vi "Replace Color.vi"(4 "Use New Fill Algorithm? (F)":bool, 5 "Swap Out White":bool, 6 "Points In":i32[][](array[numeric]), 7 "New Color":u32(colorbox), 8 "5 Pixels":i32[][](array[numeric]), 9 "Ref Color":u32, 10 "U32 color":u32[](array[numeric]), 11 "Rectangle":T1={"left"=0, "top"=0, "right"=32, "bottom"=32}) -> (3 "RGB out":u8[](array[numeric]))   [LabVIEW 2021, in "lv_icon.lvlib"]
doc: "Fill all neightbouring pixels with a certain color based on the incoming start coordinates."
uses:
  lv_icon.lvlib
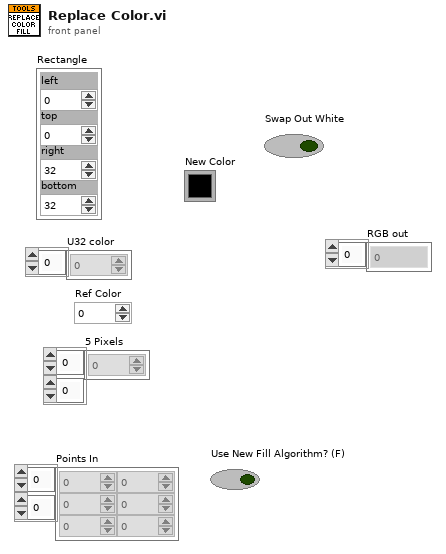
[diagram p1: front panel]
types:
  T1 = cluster{"left":i16, "top":i16, "right":i16, "bottom":i16}
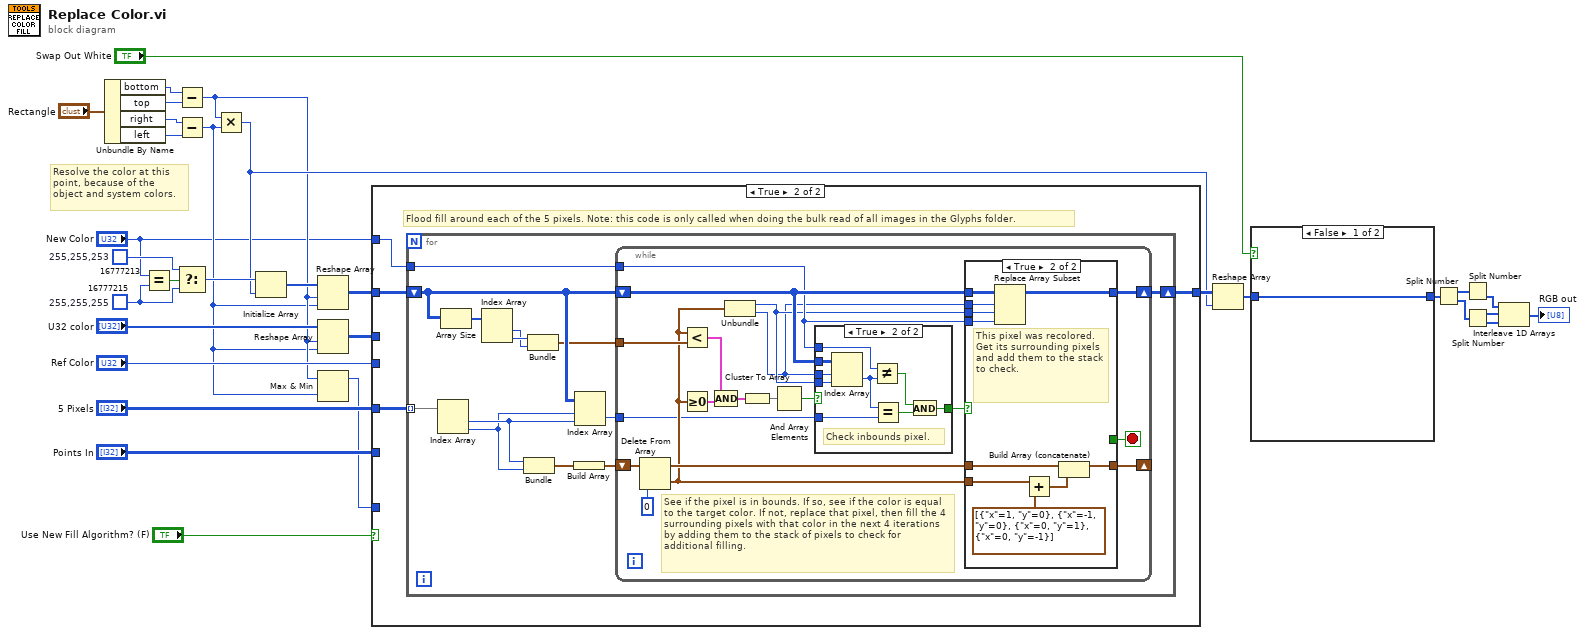
[diagram p0: block diagram]
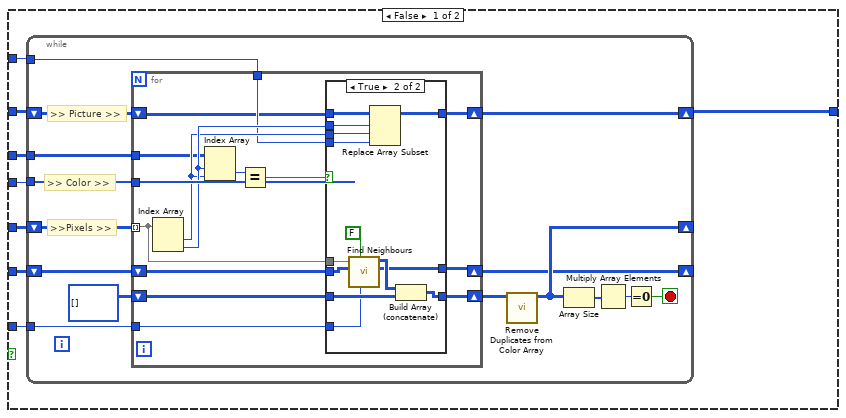
[diagram p2: hidden frame]
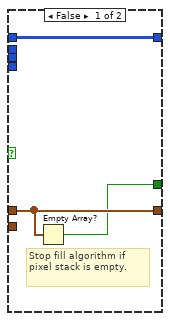
[diagram p5: hidden frame]
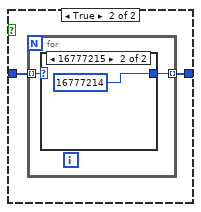
[diagram p6: hidden frame]
diagram:
  w7 = u32 16777213  # 255,255,253
  w6 = u32 16777215  # 255,255,255
  # "Resolve the color at this\npoint, because of the\nobject and system colors."
  n1 = Unbundle By Name("Rectangle") -> ("bottom"=w13:i16, "top"=w14:i16, "right"=w15:i16, "left"=w16:i16)
  n2 = Equal?(x="New Color", y=w6) -> (x = y?=w8:bool)
  n3 = Subtract(x=w13, y=w14) -> (x-y=w11:i16)
  n4 = Subtract(x=w15, y=w16) -> (x-y=w10:i16)
  n5 = Select(t=w7, s=w8, f=w6) -> (s? t:f=w18:u32)
  n6 = Multiply(x=w11, y=w10) -> (x*y=w12:i16)
  n7 = Initialize Array(w18, w12) -> (w28:u32[])
  n8 = Reshape Array(w28, w11, w10) -> (w30:u32[][])
  n9 = Reshape Array("U32 color", w11, w10) -> (w29:u32[][])
  n10 = Max & Min(x=w11, y=w10) -> (max(x,y)=w9:i16)  [unwired: 1 out]
  n11 = case shown="True" "Use New Fill Algorithm? (F)" {
    tunnel: "5 Pixels" -> [w40 w87]
    tunnel: w30 -> [w39 w90]
    tunnel: w29 -> [w38 _]
    tunnel: [w37 w89] -> w27
    tunnel: "Points In" -> [w36 _]
    tunnel: "Ref Color" -> [w35 _]
    tunnel: w9 -> [w34 _]
    tunnel: "New Color" -> [w33 w88]
    frame False {
      n12 = while {
        tunnel: w35 -> [w55]
        tunnel: w33 -> [w53]
        shift-right: [w48] -> _
        shift-left: w40 -> [w43]
        shift-right: [w41] -> w37
        shift-left: w39 -> [w47]
        tunnel: w38 -> [w46]
        shift-right: [w45] -> _
        shift-left: w36 -> [w44]
        tunnel: w34 -> [w42]
        stop <- w51 stop-if-true
        # ">> Picture >>"
        # ">>Pixels >>"
        # ">> Color >>"
        n13 = for {
          tunnel: w43 -> [w68] mode=indexing
          tunnel: w55 -> [w70]
          shift-right: [w67] -> w49
          shift-left: i32[][] [] -> [w66]
          tunnel: w53 -> [w62]
          tunnel: w46 -> [w60]
          shift-right: [w56] -> w41
          shift-left: w47 -> [w61]
          shift-right: [w58] -> w45
          shift-left: w44 -> [w59]
          tunnel: w42 -> [w57]
          n14 = Index Array(array=w68) -> (element #1=w63:i32, element #2=w64:i32)  [unwired: 2 in]
          n15 = Index Array(array=w60, index (row)=w64, index (col)=w63) -> (element=w69:u32)
          n16 = Equal?(x=w69, y=w70) -> (x = y?=w65:bool)
          n17 = case shown="True" w65 {
            tunnel: w68 -> [_ w86]
            tunnel: [w73 w84] -> w67
            tunnel: w66 -> [w73 w83]
            tunnel: w61 -> [w72 w81]
            tunnel: [w72 w80] -> w56
            tunnel: w64 -> [_ w79]
            tunnel: w63 -> [_ w78]
            tunnel: w62 -> [_ w77]
            tunnel: w59 -> [w71 w76]
            tunnel: [w71 w75] -> w58
            tunnel: w57 -> [_ w74]
            frame False {
            }
            frame True {
              n18 = call "Find Neighbours.vi"("#"=w74, "Add Start Point?"=FALSE, "Points In"=w76, "XY"=w86) -> ("Points out"=w75:i32[][], "Filtered"=w85:i32[][])  [unwired: 6 out]
              n19 = Replace Array Subset(array=w81, new element=w77, index (row)=w79, index (col)=w78) -> (w80:u32[][])
              n20 = Build Array (concatenate)(w85, w83) -> (w84:i32[][])
            }
          }
        }
        n21 = call "Remove Duplicates from Color Array.vi"("Array In"=w49) -> ("Array Out"=w48:i32[][])  [unwired: 10 out]
        n22 = Array Size(array=w48) -> (size(s)=w50:i32[])
        n23 = Multiply Array Elements(1:w50) -> (0:w52:i32)
        n24 = Equal To 0?(x=w52) -> (x = 0?=w51:bool)
      }
    }
    frame True {
      # "Flood fill around each of the 5 pixels. Note: this code is only called when doing the bulk read of all images in the Glyphs folder."
      n25 = for {
        tunnel: w88 -> [w98]
        shift-right: [w100] -> w89
        shift-left: w90 -> [w99]
        tunnel: w87 -> [w97] mode=indexing
        n26 = Index Array(array=w97) -> (element #1=w94:i32, element #2=w93:i32)  [unwired: 2 in]
        n27 = Array Size(array=w99) -> (size(s)=w101:i32[])
        n28 = Index Array(array=w101) -> (element #1=w91:i32, element #2=w92:i32)  [unwired: 2 in]
        n29 = Bundle(w94, w93) -> (w95:cluster{i32, i32})  [unwired: 1 in]
        n30 = Bundle(w92, w91) -> (w96:cluster{i32, i32})  [unwired: 1 in]
        n31 = Build Array(w95) -> (w102:cluster{i32, i32}[])
        n32 = Index Array(array=w99, index (row)=w93, index (col)=w94) -> (element=w103:u32)
        n33 = while {
          shift-right: [w122] -> w100
          shift-left: w99 -> [w120]
          shift-right: [w119] -> _
          shift-left: w102 -> [w118]
          tunnel: w103 -> [w104]
          tunnel: w96 -> [w113]
          tunnel: w98 -> [w108]
          stop <- w109 stop-if-true
          # "See if the pixel is in bounds. If so, see if the color is equal to the target color. If not, replace that pixel, then fill the 4 surrounding pixels with that color in the next 4 iterations by adding them to the stack of pixels to check for additional filling."
          n34 = Delete From Array(array=w118, index=0) -> (deleted portion=w107:cluster{i32, i32}, array with subset deleted=w117:cluster{i32, i32}[])  [unwired: 1 in]
          n35 = Less?(x=w107, y=w113) -> (x < y?=w115:cluster{bool, bool})
          n36 = Greater Or Equal To 0?(x=w107) -> (x >= 0?=w114:cluster{bool, bool})
          n37 = Compound Arithmetic op=AND(w115, w114) -> (w112:cluster{bool, bool})
          n38 = Unbundle(w107) -> (w106:i32, w105:i32)
          n39 = Cluster To Array(cluster=w112) -> (array=w111:bool[])
          n40 = And Array Elements(Boolean array=w111) -> (logical AND=w110:bool)
          n41 = case shown="True" w110 {
            selector: w110 -> [w123 _]
            tunnel: w120 -> [_ w132]
            tunnel: [w123 w130] -> w121
            tunnel: w104 -> [_ w131]
            tunnel: w108 -> [_ w124]
            tunnel: w105 -> [_ w129]
            tunnel: w106 -> [_ w128]
            frame False {
              # "Pixel out of bounds."
            }
            frame True {
              # "Check inbounds pixel."
              n42 = Index Array(array=w132, index (row)=w129, index (col)=w128) -> (element=w127:u32)
              n43 = Not Equal?(x=w124, y=w127) -> (x != y?=w125:bool)
              n44 = Equal?(x=w127, y=w131) -> (x = y?=w126:bool)
              n45 = And(x=w125, y=w126) -> (x .and. y?=w130:bool)
            }
          }
          n46 = case shown="True" w121 {
            tunnel: w120 -> [w135 w145]
            tunnel: [w135 w144] -> w122
            tunnel: w108 -> [_ w143]
            tunnel: w106 -> [_ w139]
            tunnel: w105 -> [_ w140]
            tunnel: w107 -> [_ w138]
            tunnel: w117 -> [w134 w142]
            tunnel: [w134 w141] -> w119
            tunnel: [w133 _] -> w109
            frame False {
              # "Stop fill algorithm if pixel stack is empty."
              n47 = Empty Array?(array=w134) -> (empty?=w133:bool)
            }
            frame True {
              # "This pixel was recolored. Get its surrounding pixels and add them to the stack to check."
              n48 = Replace Array Subset(array=w145, new element=w143, index (row)=w140, index (col)=w139) -> (w144:u32[][])
              n49 = Add(x=w138, y=cluster{"x":i32, "y":i32}[] [{"x"=1, "y"=0}, {"x"=-1, "y"=0}, {"x"=0, "y"=1}, {"x"=0, "y"=-1}]) -> (x+y=w137:cluster{i32, i32}[])
              n50 = Build Array (concatenate)(w142, w137) -> (w141:cluster{i32, i32}[])
            }
          }
        }
      }
    }
  }
  n51 = Reshape Array(w27, w12) -> (w3:u32[])
  n52 = case shown="False" "Swap Out White" {
    tunnel: [w146 w147] -> w4
    tunnel: w3 -> [w146 w148]
    frame False {
    }
    frame True {
      n53 = for {
        tunnel: w148 -> [w150] mode=indexing
        tunnel: [w149] -> w147 mode=indexing
        n54 = case shown="16777215" w150 {
          selector: w150 -> [w151 _]
          tunnel: [w151 u32 16777214 ("255,255,255")] -> w149
          frame Default {
          }
          frame 16777215 {
          }
        }
      }
    }
  }
  n55 = Split Number(x=w4) -> (hi(x)=w25:u16[], lo(x)=w26:u16[])
  n56 = Split Number(x=w25) -> (lo(x)=w24:u8[])  [unwired: 1 out]
  n57 = Split Number(x=w26) -> (hi(x)=w23:u8[], lo(x)=w22:u8[])
  n58 = Interleave 1D Arrays(w24, w23, w22) -> (→"RGB out":u8[])
